vi "Game 2.vi"() -> ()   [LabVIEW 2012]
uses:
  Controls/Wiimote LEDs.ctl
  Class/LV Wiimote Interface.lvclass
panel:
  out "Game Time":dbl
  in  "Min game time (s)":dbl=60.0
  out "Player 2 \nScore":dbl(slide) scale=0.0..100.0
  out "Player 1 \nScore":dbl(slide) scale=0.0..100.0
  in  "Single player?":bool
  in  "Iterations per \nSine Wave":i32=100
  in  "Restart?":bool
  in  "stop":bool
  in  "Loop Period (ms)":u32=50
  out "Waveform Chart":cluster{sgl, sgl, dbl}(graph)
  out "actual loop rate (ms)":u32
  out "error out":errorcluster
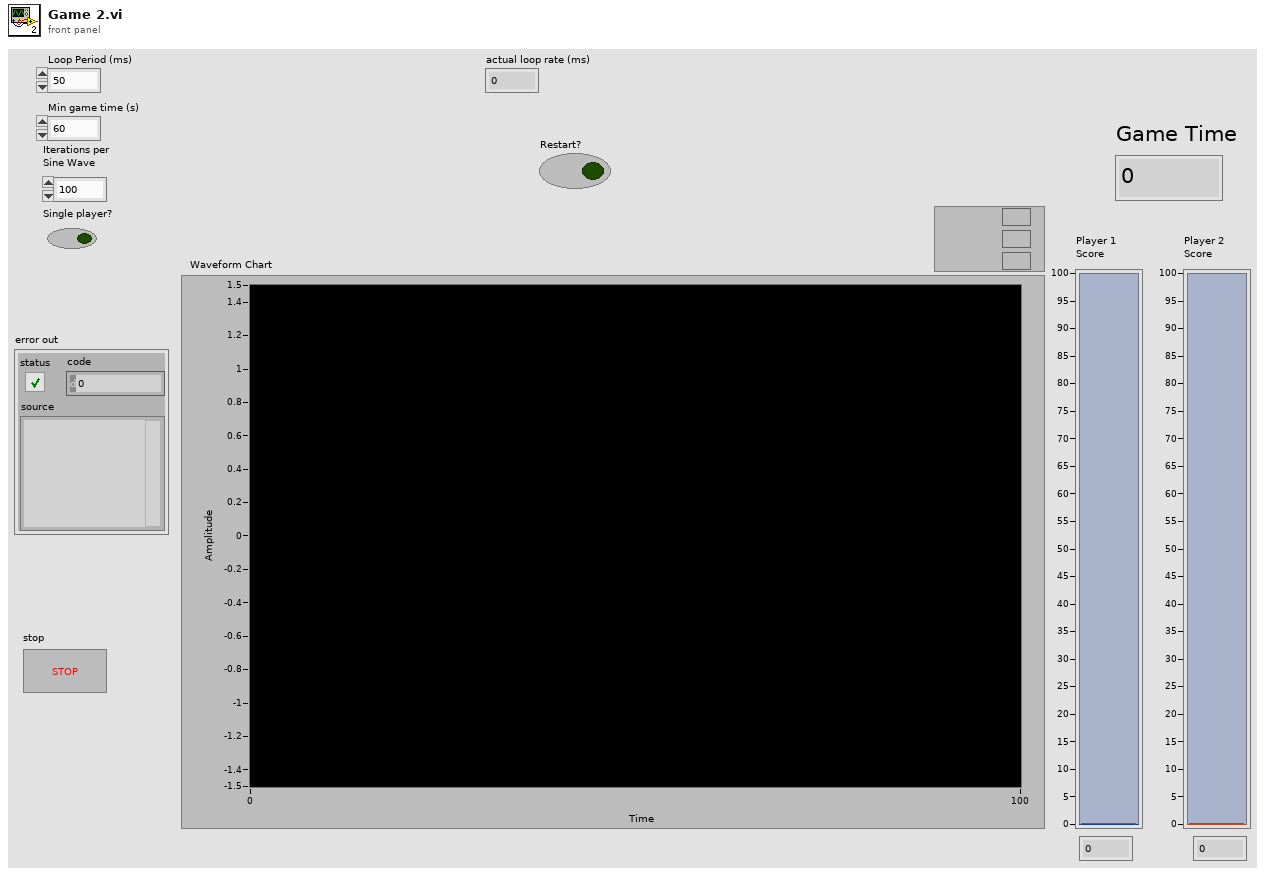
[diagram p1: front panel]
types:
  T1 = typedef "LV Wiimote Interface.lvclass/Wiimote LEDs.ctl" = cluster{"Wiimote LED":bool, "Wiimote LED 2":bool, "Wiimote LED 3":bool, "Wiimote LED 4":bool}
  T2 = typedef "LV Wiimote Interface.ctl" = refnum<class "LV Wiimote Interface.lvclass">
  T3 = typedef "LV Wiimote Interface.lvclass/XYZ Acceleration.ctl" = cluster{"X":sgl, "Y":sgl, "Z":sgl}
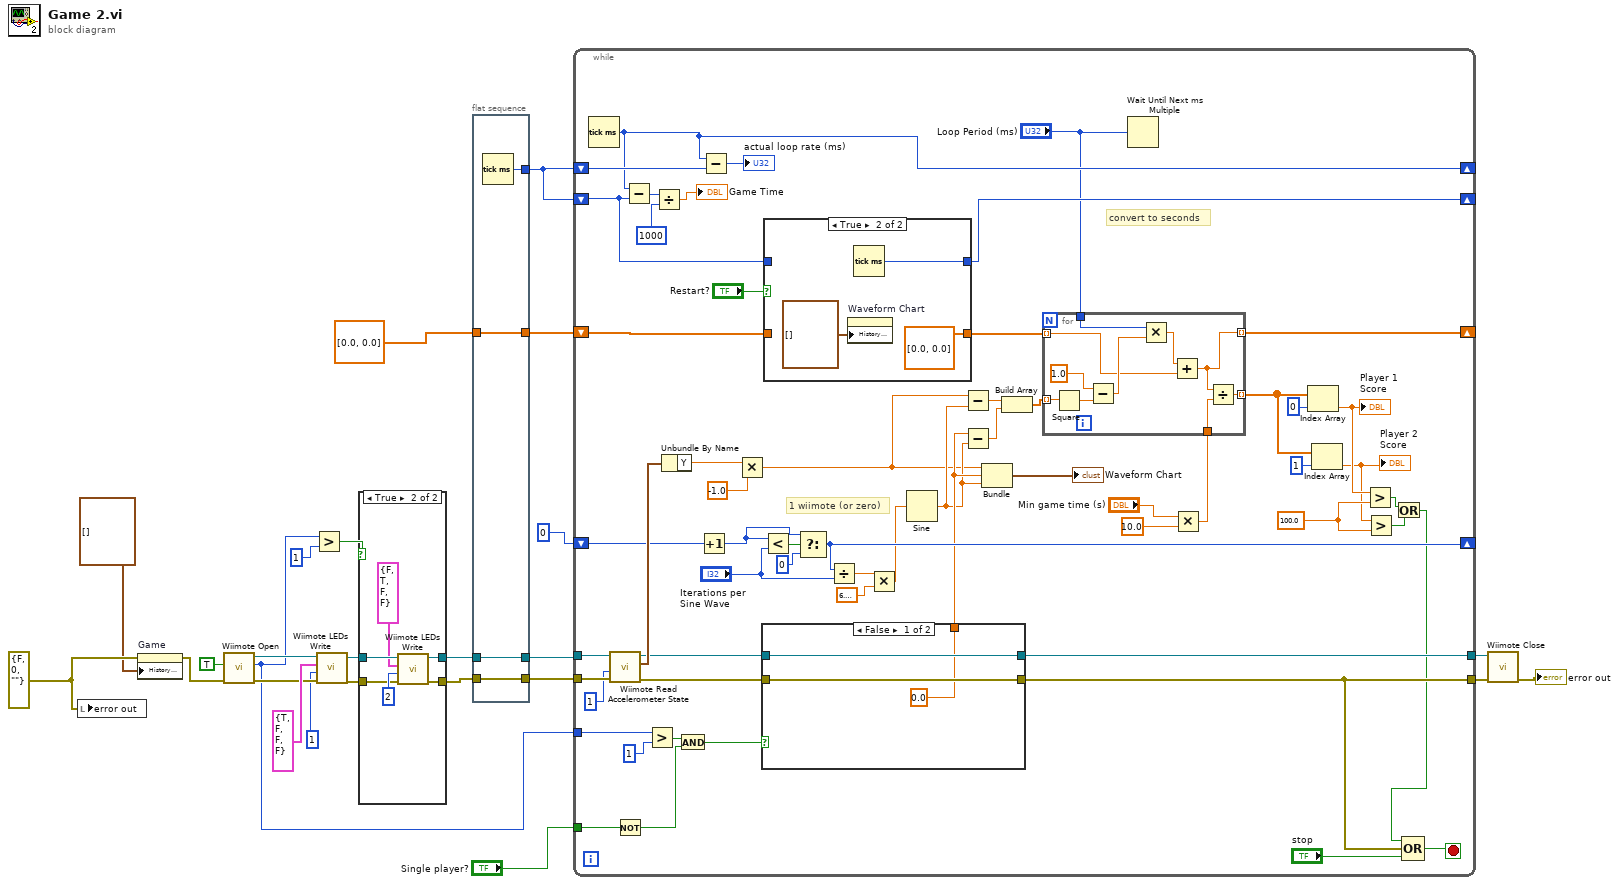
[diagram p0: block diagram]
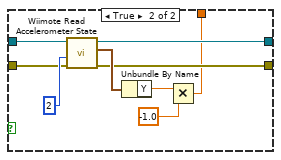
[diagram p3: hidden frame]
diagram:
  w20 = errorcluster {"status"=FALSE, "code"=0, "source"=""} ("error in (no error)")
  n1 = local write "error out"(w20) -> ()
  n2 = property on="Game" class="WFChart (strict)"(error in=w20, "History Data"=cluster{sgl, sgl, dbl}[] []) -> (error out=w19:errorcluster)  [unwired: 1 in, 1 out]
  n3 = call "Wiimote Open.vi"("error in (no error)"=w19, "Connect to all?"=TRUE) -> ("error out"=w10:errorcluster, "# Wiimotes connected"=w8:i32, "LV WiiMote Interface"=w16:T2)  [unwired: 7 in]
  n4 = Greater?(x=w8, y=1) -> (0:w13:bool)
  n5 = call "Wiimote LEDs Write.vi"("error in (no error)"=w10, "Wiimote Player #"=1, "Wiimote LEDs In"=T1 {"Wiimote LED"=TRUE, "Wiimote LED 2"=FALSE, "Wiimote LED 3"=FALSE, "Wiimote LED 4"=FALSE}, "LV WiiMote Interface In"=w16) -> ("error out"=w12:errorcluster, "LV WiiMote Interface out"=w17:T2)  [unwired: 5 in, 1 out]
  n6 = case shown="True" w13 {
    tunnel: w17 -> [w27 w33]
    tunnel: w12 -> [w26 w30]
    tunnel: [w27 w29] -> w2
    tunnel: [w26 w28] -> w11
    frame False {
    }
    frame True {
      n7 = call "Wiimote LEDs Write.vi"("error in (no error)"=w30, "Wiimote Player #"=2, "Wiimote LEDs In"=T1 {"Wiimote LED"=FALSE, "Wiimote LED 2"=TRUE, "Wiimote LED 3"=FALSE, "Wiimote LED 4"=FALSE}, "LV WiiMote Interface In"=w33) -> ("error out"=w28:errorcluster, "LV WiiMote Interface out"=w29:T2)  [unwired: 5 in, 1 out]
    }
  }
  n8 = flat-sequence {
    tunnel: [w37] -> w21
    tunnel: w11 -> [w36]
    tunnel: [w36] -> w18
    tunnel: dbl[] [0.0, 0.0] -> [w35]
    tunnel: [w35] -> w3
    tunnel: w2 -> [w34]
    tunnel: [w34] -> w1
    frame #0 {
      n9 = Tick Count (ms)() -> (millisecond timer value=w37:u32)
    }
  }
  n10 = while {
    tunnel: w1 -> [w96]
    tunnel: w18 -> [w95]
    tunnel: [w65] -> w24
    tunnel: [w50] -> w23
    shift-right: [w87] -> _
    shift-left: w21 -> [w93]
    tunnel: w8 -> [w82]
    shift-right: [w84] -> _
    shift-left: w21 -> [w85]
    shift-right: [w83] -> _
    shift-left: 0 -> [w76]
    tunnel: "Single player?" -> [w79]
    shift-right: [w59] -> _
    shift-left: w3 -> [w78]
    stop <- w52 stop-if-true
    w48 = 100.0 ("x")
    # "1 wiimote (or zero)"
    # "convert to seconds"
    n11 = Tick Count (ms)() -> (millisecond timer value=w87:u32)
    n12 = call "Wiimote Read Accelerometer State.vi"("error in (no error)"=w95, "Wiimote Player #"=1, "LV WiiMote Interface In"=w96) -> ("error out"=w68:errorcluster, "XYZ Acceleration"=w89:T3, "LV WiiMote Interface out"=w66:T2)  [unwired: 6 in]
    n13 = Not(x=w79) -> (.not. x?=w80:bool)
    n14 = Subtract(x=w87, y=w85) -> (x-y=w43:u32)
    n15 = Greater?(x=w82, y=1) -> (0:w81:bool)
    n16 = Divide(x=w43, y=u32 1000) -> (x/y=→"Game Time":dbl)
    n17 = Unbundle By Name(w89) -> ("Y"=w88:sgl)
    n18 = And(x=w81, y=w80) -> (x .and. y?=w67:bool)
    n19 = Increment(x=w76) -> (x+1=w74:i32)
    n20 = Subtract(x=w87, y=w93) -> (x-y=→"actual loop rate (ms)":u32)
    n21 = Multiply(x=w88, y=sgl -1.0) -> (x*y=w38:sgl)
    n22 = case shown="False" w67 {
      tunnel: w68 -> [w109 w113]
      tunnel: w66 -> [w108 w114]
      tunnel: [w108 w112] -> w65
      tunnel: [w109 w111] -> w50
      tunnel: [sgl 0.0 w110] -> w63
      frame False {
      }
      frame True {
        n23 = call "Wiimote Read Accelerometer State.vi"("error in (no error)"=w113, "Wiimote Player #"=2, "LV WiiMote Interface In"=w114) -> ("error out"=w111:errorcluster, "XYZ Acceleration"=w115:T3, "LV WiiMote Interface out"=w112:T2)  [unwired: 6 in]
        n24 = Unbundle By Name(w115) -> ("Y"=w116:sgl)
        n25 = Multiply(x=w116, y=sgl -1.0) -> (x*y=w110:sgl)
      }
    }
    n26 = Less?(x=w74, y="Iterations per \nSine Wave") -> (x < y?=w75:bool)
    n27 = case shown="True" "Restart?" {
      tunnel: w85 -> [w120 _]
      tunnel: [w120 w123] -> w84
      tunnel: [w119 dbl[] [0.0, 0.0]] -> w77
      tunnel: w78 -> [w119 _]
      frame False {
      }
      frame True {
        n28 = property on="Waveform Chart" class="WFChart (strict)"("History Data"=cluster{sgl, sgl, dbl}[] []) -> ()  [unwired: 2 in, 2 out]
        n29 = Tick Count (ms)() -> (millisecond timer value=w123:u32)
      }
    }
    n30 = Select(t=w74, s=w75, f=0) -> (s? t:f=w83:i32)
    n31 = Divide(x=w83, y="Iterations per \nSine Wave") -> (x/y=w72:dbl)
    n32 = Multiply(x=w72, y=6.283185307179586) -> (x*y=w69:dbl)
    n33 = Sine(x=w69) -> (sin(x)=w39:dbl)
    n34 = Subtract(x=w38, y=w39) -> (x-y=w61:dbl)
    n35 = Subtract(x=w63, y=w39) -> (x-y=w62:dbl)
    n36 = Bundle(w38, w63, w39) -> (→"Waveform Chart":cluster{sgl, sgl, dbl})  [unwired: 1 in]
    n37 = Build Array(w61, w62) -> (w60:dbl[])
    n38 = Wait Until Next ms Multiple(millisecond multiple="Loop Period (ms)") -> ()  [unwired: 1 out]
    n39 = Multiply(x="Min game time (s)", y=10.0) -> (x*y=w40:dbl)
    n40 = for {
      tunnel: "Loop Period (ms)" -> [w105]
      tunnel: w77 -> [w102] mode=indexing
      tunnel: w60 -> [w100] mode=indexing
      tunnel: [w99] -> w59 mode=indexing
      tunnel: [w98] -> w57 mode=indexing
      tunnel: w40 -> [w97]
      n41 = Square(x=w100) -> (x^2=w101:dbl)
      n42 = Subtract(x=1.0, y=w101) -> (x-y=w103:dbl)
      n43 = Multiply(x=w105, y=w103) -> (x*y=w104:dbl)
      n44 = Add(x=w104, y=w102) -> (x+y=w99:dbl)
      n45 = Divide(x=w99, y=w97) -> (x/y=w98:dbl)
    }
    n46 = Index Array(array=w57, index=0) -> (element=w55:dbl)
    "Player 1 \nScore" <- w55
    n47 = Index Array(array=w57, index=1) -> (element=w47:dbl)
    "Player 2 \nScore" <- w47
    n48 = Greater?(x=w55, y=w48) -> (0:w54:bool)
    n49 = Greater?(x=w47, y=w48) -> (0:w53:bool)
    n50 = Or(x=w54, y=w53) -> (x .or. y?=w49:bool)
    n51 = Compound Arithmetic op=OR(w49, w50, "stop") -> (w52:bool)
  }
  n52 = call "Wiimote Close.vi"("error in (no error)"=w23, "LV WiiMote Interface"=w24) -> ("error out"=→"error out":errorcluster)  [unwired: 9 in]
